vi "FlowChart Edit All.vi"(10 "Name":string, 11 "Identifier In":string[](array[string])) -> (2 "OK？":bool, 3 "Identifiers Out":string[](array[string]))   [LabVIEW 2020]
uses:
  <vilib>/Utility/miscctls.llb/LVRowAndColumnUnsignedTypeDef.ctl
  bf13b16f-8a27-41fb-9ad8-d28ab69cb5d9.vi
panel:
  in  "Group":u16(ring) items=["", "故障报警", "WEB", "设备安全状态", "氢气路", "CVM", "电子负载", "电子负载参数", "氮气路", "空气路", "去离子水", "系统计算数据", "电堆热管理模块"]
  in  "Serrch Info":string
  in  "Search":bool
  in  "Selected Data":i32[](listbox) caption="已选择数据"
  in  "Add":bool
  in  "Delete":bool
  in  "All Data":i32[](listbox) caption="全部数据"
  in  "OK":bool
  in  "Cancel":bool
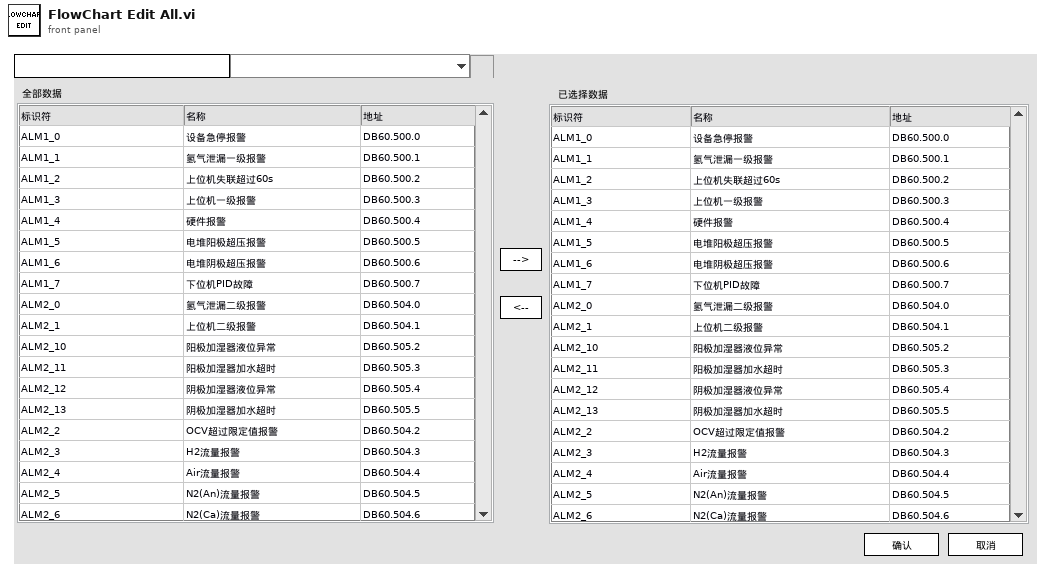
[diagram p1: front panel]
types:
  T1 = typedef "LVRowAndColumnUnsignedTypeDef.ctl" = cluster{"Row":u32, "Column":u32}
  T2 = cluster{"All Data":string[][], "Selected Data":string[][], "Group":string[]}
  T3 = enum32{"Invalid", "Default", "Floating", "Floating/Auto-Hide", "Modal"}
  T4 = typedef "SDQ Data Type.ctl" = cluster{"CAN Length":string, "CAN Name":string, "CAN ID":string, "CAN Type":string, "Test Item":string, "Byte Order":string, "Instruction":string, "Control Type":string, "Group":string, "Offset":dbl, "Coefficient":dbl, "Write Enable":bool, "Lable Type":string, "Key?":string, "Set Value":string, "Upper":dbl, "Lower":dbl, "Unit":string, "Formula":string, "Test Item Type":string, "Length":i32, "Address":string, "Name":string, "Identifier":string, "Data Type":string, "Enumerate?":string, "Enumerate List":string, "Data":string, "Source":string}
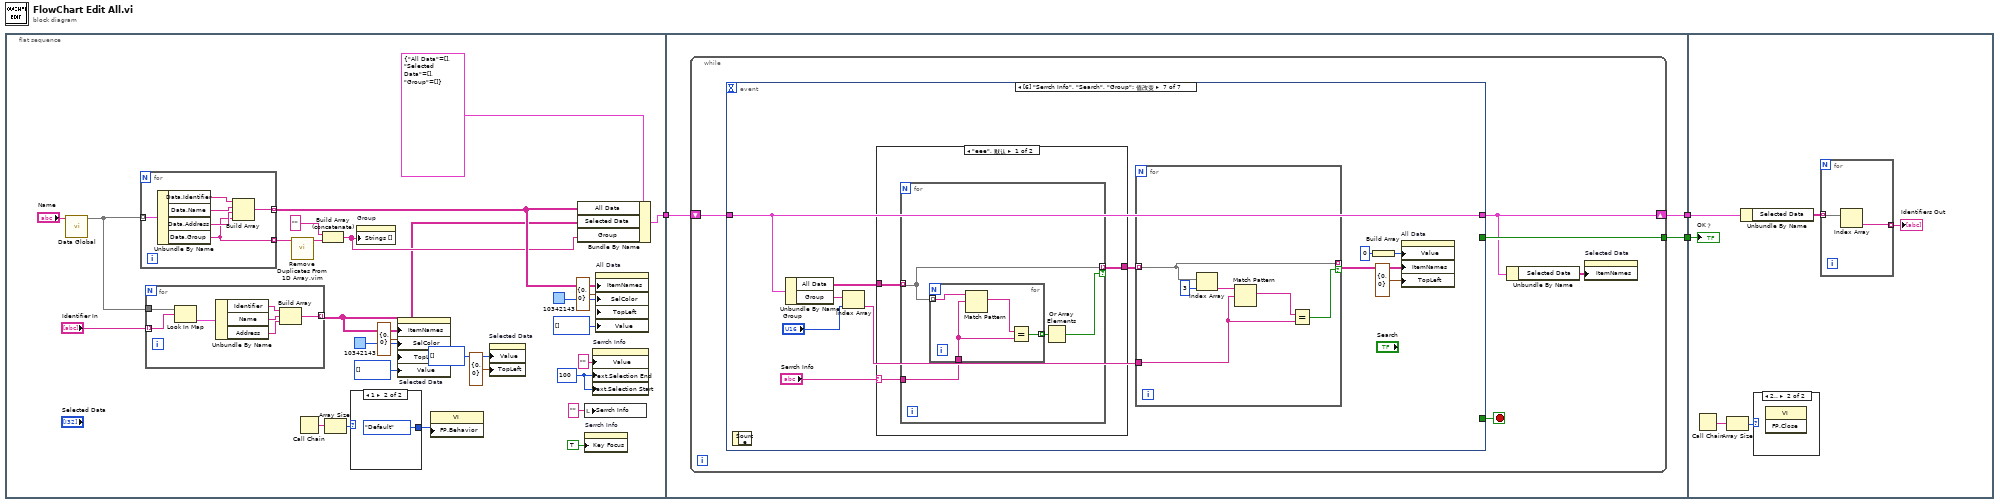
[diagram p0: block diagram]
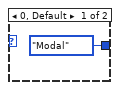
[diagram p2: hidden frame]
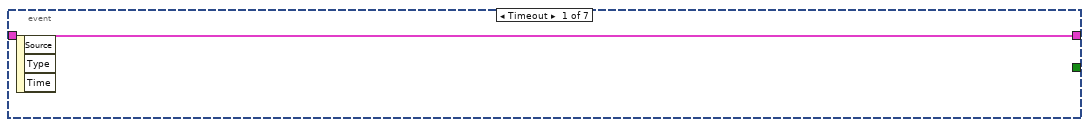
[diagram p3: hidden frame]
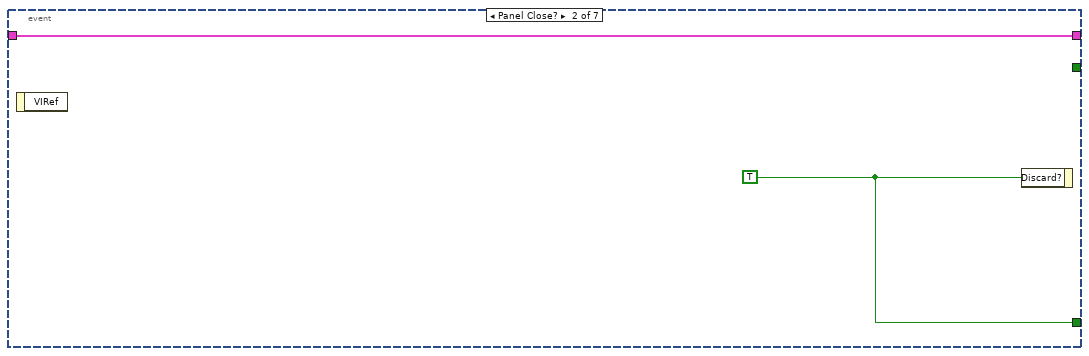
[diagram p4: hidden frame]
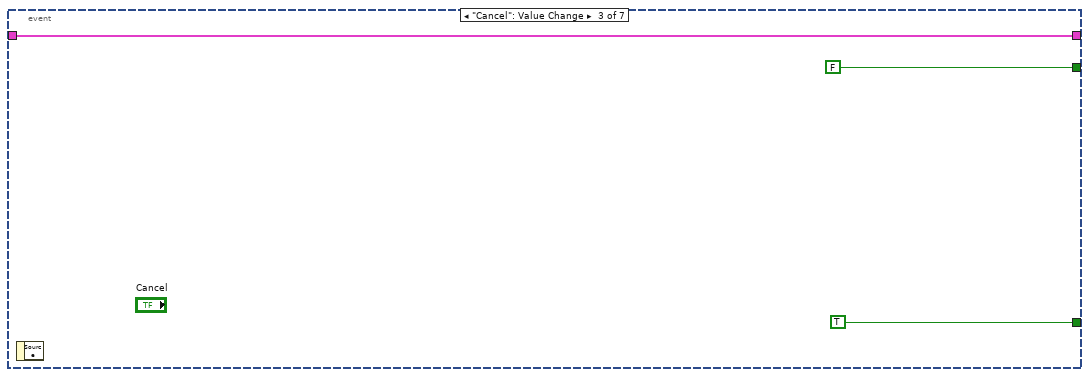
[diagram p5: hidden frame]
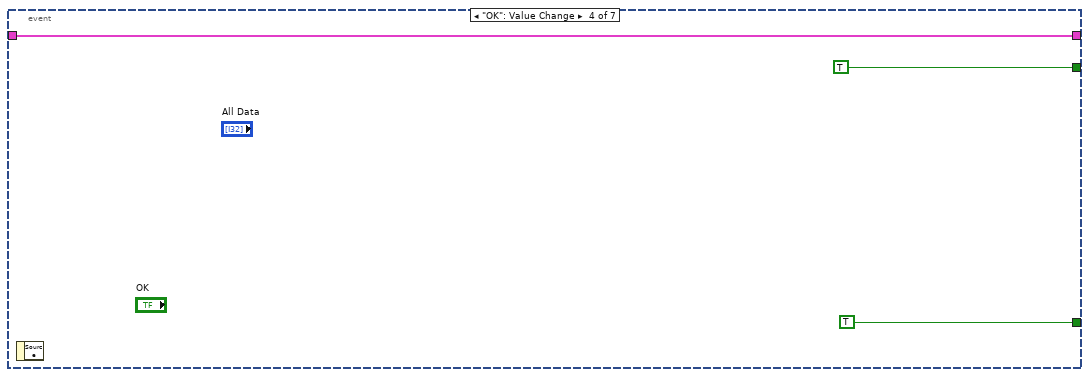
[diagram p6: hidden frame]
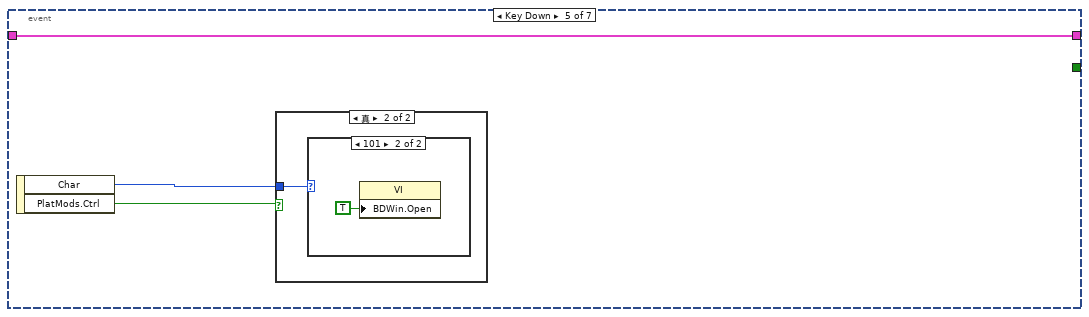
[diagram p7: hidden frame]
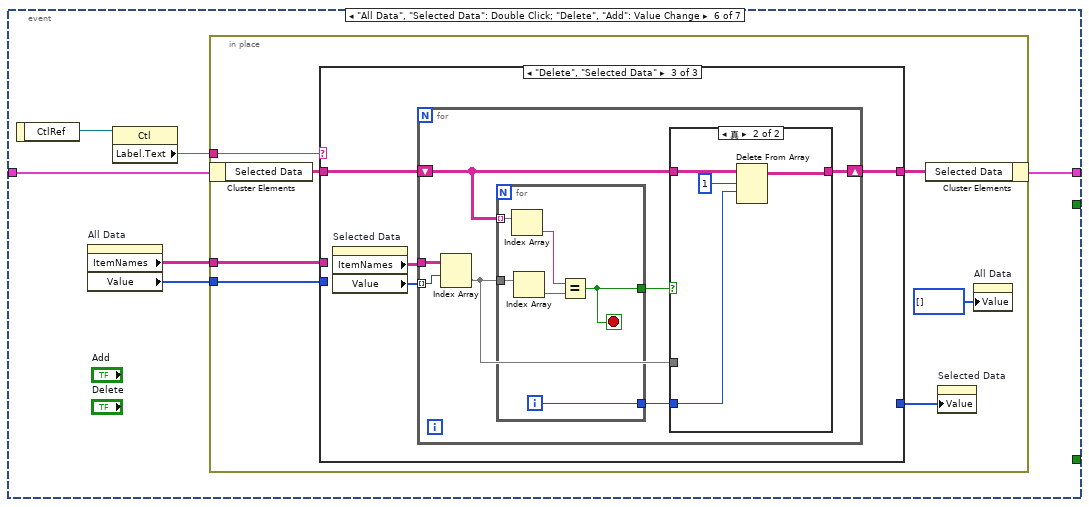
[diagram p10: hidden frame]
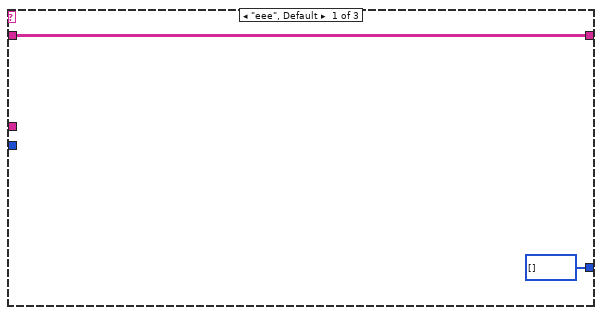
[diagram p11: hidden frame]
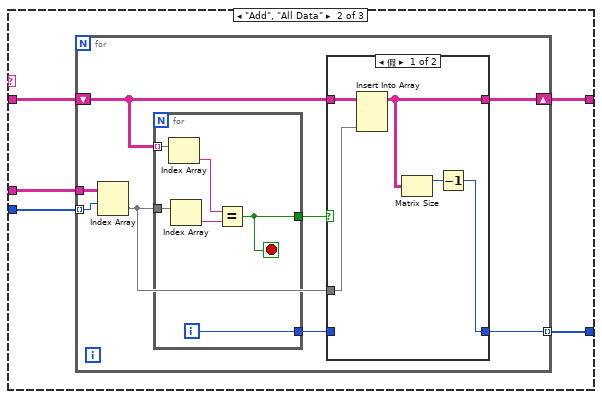
[diagram p12: hidden frame]
diagram:
  n1 = flat-sequence {
    tunnel: [w16] -> w2
    tunnel: [w47] -> w3
    tunnel: w2 -> [w46]
    tunnel: [w45] -> w1
    tunnel: w3 -> [w164]
    tunnel: w1 -> [w161]
    frame #0 {
      w26 = u32 100 ("文本.选择区域:末尾")
      n2 = call "Data Global.vi"("Name"="Name") -> ("Data Out"=w5:map{string, T4})  [unwired: 7 in, 3 out]
      n3 = for {
        tunnel: w5 -> [w44] mode=indexing
        tunnel: [w41] -> w17 mode=indexing
        tunnel: [w39] -> w21 mode=indexing
        n4 = Unbundle By Name(w44) -> ("Data.Identifier"=w40:string, "Data.Name"=w43:string, "Data.Address"=w42:string, "Data.Group"=w39:string)
        n5 = Build Array(w40, w43, w42, w39) -> (w41:string[])
      }
      n6 = for {
        tunnel: "Identifier In" -> [w34] mode=indexing
        tunnel: w5 -> [w35]
        tunnel: [w32] -> w7 mode=indexing
        n7 = Look In Map(map=w35, key=w34) -> (value=w33:T4)  [unwired: 1 in, 1 out]
        n8 = Unbundle By Name(w33) -> ("Identifier"=w36:string, "Name"=w37:string, "Address"=w38:string)
        n9 = Build Array(w36, w37, w38) -> (w32:string[])
      }
      n10 = call "Remove Duplicates From 1D Array.vim"("array"=w21) -> ("array with duplicates removed"=w20:string[])  [unwired: 10 in]
      n11 = Call Chain() -> (call chain=w14:string[])
      n12 = Build Array (concatenate)("", w20) -> (w11:string[])
      n13 = Array Size(array=w14) -> (size(s)=w15:i32)
      n14 = case shown="1" w15 {
        tunnel: [T3."Modal" ("前面板窗口:动作") T3."Default" ("前面板窗口:动作")] -> w10
        frame 0, Default {
        }
        frame 1 {
        }
      }
      n15 = property on="Group" class="Ring (严格)"("Strings []"=w11) -> ()  [unwired: 2 in, 2 out]
      n16 = property on="Selected Data" class="MCListbox (严格)"("ItemNames"=w7, "SelColor"=u32 10342143 ("选择颜色"), "TopLeft"=T1 {"Row"=0, "Column"=0} ("左上可见单元格"), "Value"=i32[] [] ("Selected Data")) -> ()  [unwired: 2 in, 2 out]
      n17 = property class="VI"("FP.Behavior"=w10) -> ()  [unwired: 2 in, 2 out]
      n18 = property on="Selected Data" class="MCListbox (严格)"("Value"=i32[] [] ("Selected Data"), "TopLeft"=T1 {"Row"=0, "Column"=0} ("左上可见单元格")) -> ()  [unwired: 2 in, 2 out]
      n19 = Bundle By Name(cluster=T2 {"All Data"=[], "Selected Data"=[], "Group"=[]}, "All Data"=w17, "Selected Data"=w7, "Group"=w11) -> (w16:T2)
      n20 = local write "Serrch Info"("" ("Serrch Info")) -> ()
      n21 = property on="Serrch Info" class="Str"("Key Focus"=TRUE ("键选中")) -> ()  [unwired: 2 in, 2 out]
      n22 = property on="Serrch Info" class="Str"("Value"="" ("Serrch Info"), "Text.Selection End"=w26, "Text.Selection Start"=w26) -> ()  [unwired: 2 in, 2 out]
      n23 = property on="All Data" class="MCListbox (严格)"("ItemNames"=w17, "SelColor"=u32 10342143 ("选择颜色"), "TopLeft"=T1 {"Row"=0, "Column"=0} ("左上可见单元格"), "Value"=i32[] [] ("Data List")) -> ()  [unwired: 2 in, 2 out]
    }
    frame #1 {
      n24 = while {
        tunnel: [w51] -> w47
        shift-right: [w49] -> w45
        shift-left: w46 -> [w50]
        stop <- w52 stop-if-true
        n25 = event shown="[6] \"Serrch Info\", \"Search\", \"Group\": 值改变" {
          selector: _ -> [_ _ _ _ _ _ _]
          dyn-events: _ -> [_ _ _ _ _ _ _]
          timeout: _ -> [_ _ _ _ _ _ _]
          tunnel: [_ w55 TRUE ("放弃？") TRUE ("放弃？") _ _ _] -> w52
          tunnel: [_ _ FALSE TRUE _ _ _] -> w51
          tunnel: w50 -> [w53 w54 w56 w59 w64 w72 w136]
          tunnel: [w53 w54 w56 w59 w64 w71 w136] -> w49
          event Timeout {
            n26 = event-data() -> ()  [unwired: 1 in, 3 out]
          }
          event Panel Close? {
            w55 = TRUE ("放弃？")
            n27 = event-data() -> ()  [unwired: 1 in, 1 out]
            n28 = event-data("Discard?"=w55) -> ()  [unwired: 1 in, 1 out]
          }
          event "Cancel": Value Change {
            n29 = event-data() -> ()  [unwired: 1 in, 1 out]
          }
          event "OK": Value Change {
            n30 = event-data() -> ()  [unwired: 1 in, 1 out]
          }
          event Key Down {
            n31 = event-data() -> ("Char"=w62:i16, "PlatMods.Ctrl"=w63:bool)  [unwired: 1 in]
            n32 = case shown="真" w63 {
              tunnel: w62 -> [_ w65]
              frame False {
              }
              frame True {
                n33 = case shown="101" w65 {
                  frame 0, Default {
                  }
                  frame 101 {
                    n34 = property class="VI"("BDWin.Open"=TRUE ("程序框图窗口:打开")) -> ()  [unwired: 2 in, 2 out]
                  }
                }
              }
            }
          }
          event "All Data", "Selected Data": Double Click; "Delete", "Add": Value Change {
            n35 = event-data() -> ("CtlRef"=w70:refnum<vi>)  [unwired: 1 in]
            n36 = property on="All Data" class="MCListbox (严格)"() -> ("ItemNames"=w67:string[][], "Value"=w68:i32[])  [unwired: 2 in, 2 out]
            n37 = property class="Ctl"(reference=w70) -> ("Label.Text"=w69:string)  [unwired: 1 in, 2 out]
            n38 = in-place {
              in-place-border: w69 -> [w74]
              in-place-border: w68 -> [w76]
              in-place-border: w67 -> [w75]
              n39 = in-place-cluster #1(w72) -> ("Selected Data"=w79:string[][])
              n40 = case shown="\"Delete\", \"Selected Data\"" w74 {
                tunnel: w79 -> [w81 w86 w111]
                tunnel: [w81 w85 w110] -> w78
                tunnel: [i32[] [] w84 _] -> w77
                tunnel: w76 -> [_ w82 _]
                tunnel: w75 -> [_ w83 _]
                frame "eee", Default {
                }
                frame "Add", "All Data" {
                  n41 = for {
                    tunnel: [w90] -> w84 mode=indexing
                    tunnel: w83 -> [w89]
                    tunnel: w82 -> [w87] mode=indexing
                    shift-right: [w92] -> w85
                    shift-left: w86 -> [w94]
                    n42 = Index Array(array=w89, index (row)=w87) -> (element=w88:string[])  [unwired: 1 in]
                    n43 = for {
                      tunnel: w88 -> [w106]
                      tunnel: w94 -> [w107] mode=indexing
                      tunnel: [w103] -> w93
                      tunnel: [w102] -> w91
                      i -> [w102]
                      stop <- w103 stop-if-true
                      n44 = Index Array(array=w107) -> (element=w105:string)  [unwired: 1 in]
                      n45 = Index Array(array=w106) -> (element=w104:string)  [unwired: 1 in]
                      n46 = Equal?(x=w105, y=w104) -> (x = y?=w103:bool)
                    }
                    n47 = case shown="假" w93 {
                      tunnel: w94 -> [w99 w101]
                      tunnel: [w96 w101] -> w92
                      tunnel: w88 -> [w98 _]
                      tunnel: w91 -> [_ w100]
                      tunnel: [w95 w100] -> w90
                      frame False {
                        n48 = Insert Into Array(array=w99, new element=w98) -> (w96:string[][])  [unwired: 2 in]
                        n49 = Matrix Size(0:w96) -> (1:w97:i32)  [unwired: 1 out]
                        n50 = Decrement(x=w97) -> (x-1=w95:i32)
                      }
                      frame True {
                      }
                    }
                  }
                }
                frame "Delete", "Selected Data" {
                  n51 = property on="Selected Data" class="MCListbox (严格)"() -> ("ItemNames"=w109:string[][], "Value"=w108:i32[])  [unwired: 2 in, 2 out]
                  n52 = for {
                    tunnel: w109 -> [w114]
                    shift-right: [w116] -> w110
                    shift-left: w111 -> [w118]
                    tunnel: w108 -> [w112] mode=indexing
                    n53 = Index Array(array=w114, index (row)=w112) -> (element=w113:string[])  [unwired: 1 in]
                    n54 = for {
                      tunnel: w113 -> [w128]
                      tunnel: w118 -> [w129] mode=indexing
                      tunnel: [w125] -> w117
                      tunnel: [w124] -> w115
                      i -> [w124]
                      stop <- w125 stop-if-true
                      n55 = Index Array(array=w129) -> (element=w127:string)  [unwired: 1 in]
                      n56 = Index Array(array=w128) -> (element=w126:string)  [unwired: 1 in]
                      n57 = Equal?(x=w127, y=w126) -> (x = y?=w125:bool)
                    }
                    n58 = case shown="真" w117 {
                      tunnel: w118 -> [w119 w123]
                      tunnel: [w119 w122] -> w116
                      tunnel: w113 -> [_ _]
                      tunnel: w115 -> [_ w120]
                      frame False {
                      }
                      frame True {
                        n59 = Delete From Array(array=w123, length=1 ("长度"), index (row)=w120) -> (array with subset deleted=w122:string[][])  [unwired: 1 in, 1 out]
                      }
                    }
                  }
                }
              }
              n60 = in-place-cluster #1("Selected Data"=w78) -> (w71:T2)
              n61 = property on="Selected Data" class="MCListbox (严格)"("Value"=w77) -> ()  [unwired: 2 in, 2 out]
              n62 = property on="All Data" class="MCListbox (严格)"("Value"=i32[] [] ("All Data")) -> ()  [unwired: 2 in, 2 out]
            }
          }
          event "Serrch Info", "Search", "Group": Value Change {
            n63 = event-data() -> ()  [unwired: 1 in, 1 out]
            n64 = Unbundle By Name(w136) -> ("All Data"=w135:string[][], "Group"=w134:string[])
            n65 = Index Array(array=w134, index="Group") -> (element=w130:string)
            n66 = case shown="\"eee\", 默认" "Serrch Info" {
              selector: "Serrch Info" -> [w148 _]
              tunnel: w135 -> [w149 w158]
              tunnel: [w147 w158] -> w132
              frame "eee", Default {
                n67 = for {
                  tunnel: w149 -> [w151] mode=indexing
                  tunnel: w148 -> [w153]
                  tunnel: [w151] -> w147 mode=indexing if=w150
                  n68 = for {
                    tunnel: w153 -> [w156]
                    tunnel: [w155] -> w152 mode=indexing
                    tunnel: w151 -> [w154] mode=indexing
                    n69 = Match Pattern(string=w154, regular expression=w156) -> (match substring=w157:string)  [unwired: 1 in, 3 out]
                    n70 = Equal?(x=w157, y=w156) -> (x = y?=w155:bool)
                  }
                  n71 = Or Array Elements(Boolean array=w152) -> (logical OR=w150:bool)
                }
              }
              frame "" {
              }
            }
            n72 = for {
              tunnel: w132 -> [w143] mode=indexing
              tunnel: w130 -> [w144]
              tunnel: [w143] -> w131 mode=indexing if=w142
              n73 = Index Array(array=w143, index=3 ("索引")) -> (element=w146:string)
              n74 = Match Pattern(string=w146, regular expression=w144) -> (match substring=w145:string)  [unwired: 1 in, 3 out]
              n75 = Equal?(x=w145, y=w144) -> (x = y?=w142:bool)
            }
            n76 = Build Array(0 ("Data List")) -> (w137:i32[])
            n77 = property on="All Data" class="MCListbox (严格)"("Value"=w137, "ItemNames"=w131, "TopLeft"=T1 {"Row"=0, "Column"=0} ("左上可见单元格")) -> ()  [unwired: 2 in, 2 out]
          }
        }
        n78 = Unbundle By Name(w49) -> ("Selected Data"=w48:string[][])
        n79 = property on="Selected Data" class="MCListbox (严格)"("ItemNames"=w48) -> ()  [unwired: 2 in, 2 out]
      }
    }
    frame #2 {
      n80 = Call Chain() -> (call chain=w163:string[])
      n81 = Array Size(array=w163) -> (size(s)=w162:i32)
      n82 = Unbundle By Name(w161) -> ("Selected Data"=w160:string[][])
      n83 = case shown="2.." w162 {
        frame 0, Default {
        }
        frame 2.. {
          n84 = invoke class="VI" method="FP.Close"() -> ()  [unwired: 3 in, 3 out]
        }
      }
      n85 = for {
        tunnel: w160 -> [w166] mode=indexing
        tunnel: [w165] -> w159 mode=indexing
        n86 = Index Array(array=w166) -> (element=w165:string)  [unwired: 1 in]
      }
      "Identifiers Out" <- w159
      "OK？" <- w164
    }
  }
